vi "InitSyntaxColoring.vi"(11 "Scintilla":refnum<k24>) -> (3 "Scintilla":refnum<k24>)   [LabVIEW 2018]
uses:
  ScintillaNET.dll
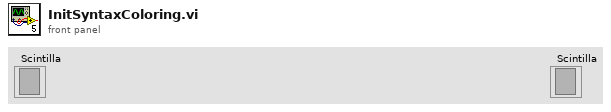
[diagram p1: front panel]
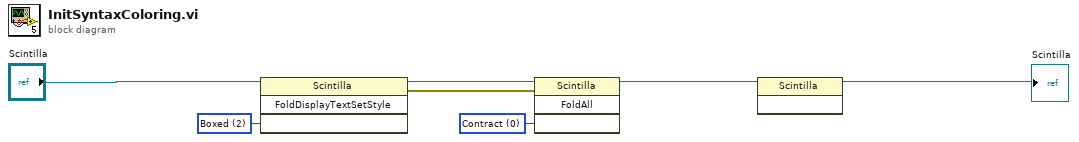
[diagram p0: block diagram]
diagram:
  w3 = 0 items=["Contract", "Expand", "Toggle"] ("action")
  w6 = 2 items=["Hidden", "Standard", "Boxed"] ("style")
  n1 = invoke on="调用节点" class="Scintilla" method="FoldDisplayTextSetStyle"(reference="Scintilla", "style"=w6) -> (reference out=w5:refnum<k24>, error out=w2:errorcluster)  [unwired: 2 in, 2 out]
  n2 = invoke on="调用节点" class="Scintilla" method="FoldAll"(reference=w5, error in=w2, "action"=w3) -> (reference out=w4:refnum<k24>)  [unwired: 1 in, 3 out]
  n3 = invoke on="调用节点" class="Scintilla" method=#-1(reference=w4) -> (reference out=→"Scintilla":refnum<k24>)  [unwired: 2 in, 2 out]
